vi "ShowMSStatus.vi"() -> ()   [LabVIEW 2015]
doc: "Use this template to create an application that executes until you click the Stop button. Unlike the Single Loop Application VI that uses polling, this VI uses the Event structure."
uses:
  _Server Global.vi
  Configuration/_Global Configuration.vi
panel:
  in  "Calibration":bool
  in  "ContactClosures":bool
  out "HideBox":bool
  in  "User Command":u16(ring)=7 items=["Start Run"=3, "Start Actual Run"=4, "Stop Run"=5, "Runtime Update"=6, "Get Data"=7, "Get Status"=8, "Get Table"=9, "Adv. Set Table"=10, "Get Configuration"=11, "Get Memory Map"=13, "Read ADC"=14, "Adv. Set Oscillator"=15, "Adv. Reboot Firmware"=16, "Adv. Backup Firmware"=17, "Adv. Update Firmware"=18, "Auxiliary Update"=19, "System Status"=20, "Start System"=21, "Shutdown System"=22, "Start LC Equilibration"=23, "Get LC Status"=24, "Get LC Configuration"=25, "Get LC Method Contents"=26, "Rinse Autosampler"=27, "Pump OnOff"=28, "Oven OnOff"=29, "Get LC Error"=30, "Clear LC Error"=31, "Set LC Input Logic"=32, "Set LC Hold Logic"=33, "Connect LC"=35, "Disconnect LC"=36]
  out "Corona Discharge:":sgl format="%.1f"
  out "ElectroSpray V2:":sgl
  out "ElectroSpray V1:":sgl
  in  "UpdateDisplay":bool
  out "Heating Gas 2:":sgl
  out "Heating Gas 1:":sgl
  out "Nebulizer Gas 1:":sgl
  out "Nebulizer Gas 2:":sgl
  out "Collision Pressure:":sgl format="%.1f"
  out "Dry Gas:":sgl
  out "Exhaust:":sgl
  out "Pump Speed:":sgl
  out "Exhaust OK":bool
  out "CurGas OK":bool
  out "Pump OK":bool
  out "Interlock OK":bool
  out "Vac. Pressure:":sgl format="%.2e"
  out "HSID Temp:":sgl
  out "Source 2 Temp:":sgl
  out "Source 2 Type:":i8(ring) items=["None", "ESI", "APCI", "APPI", "MicroSpray"]
  out "Source 1 Temp:":sgl
  out "Source 1 Type:":i8(ring) items=["None", "ESI", "APCI", "APPI", "MicroSpray"]
  out "Scans":i32 caption="Data Queue"
  out "Connected":bool=TRUE
  out "Error":string
  out "Data":string
  out "Ready":bool=TRUE
  in  "Message":string="<Method>\n  1\t0\t0\n  <Experiment>\n    1\t0\t0\t200\t0\t100\t1\t0\n    <MassRange>\n      200.000000\t400\t0.100000\t2000\t0.1\t0\n      <ParamTable/>\n    </MassRange>\n  </Experiment>\n</Method>"
  out "Data Queue":i32
  out "Busy":bool
  out "Locked":bool
  # "Source 1"
  # "Common Interface"
  # "Source 2"
  # "Other Status"
  # "Torr"
  # "Interlocks:"
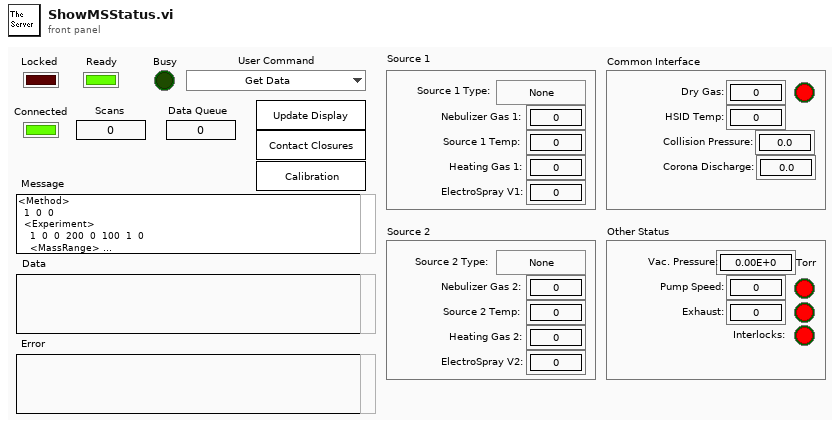
[diagram p1: front panel]
types:
  T1 = typedef "_Brief Status.ctl" = cluster{"Source 1 Type: ":T2, "Nebulizer Gas 1:":sgl, "Probe Temp 1: ":sgl, "Heating Gas 1:":sgl, "Source 2 Type:  ":T2, "Nebulizer Gas 2:":sgl, "Probe Temp 2: ":sgl, "Heating Gas 2:":sgl, "Dry Gas:":sgl, "HSID Temp:  ":sgl, "Collision Gas:":sgl, "Vac. Pressure: ":sgl, "Pump Speed:":sgl, "Exhaust:":sgl, "Interlock OK":bool, "CurGas OK":bool, "Pump OK":bool, "Exhaust OK":bool, "Event":string, "Corona Discharge:":sgl, "Source 1 Voltage:":sgl, "Source 2 Voltage:":sgl}
  T2 = typedef "_Source Type.ctl" = i8
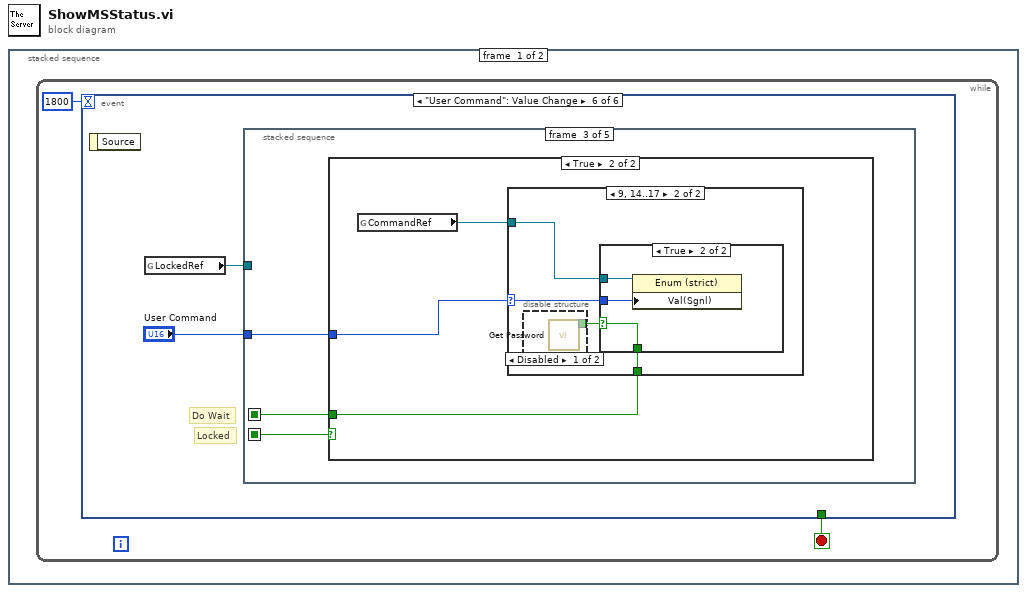
[diagram p0: block diagram]
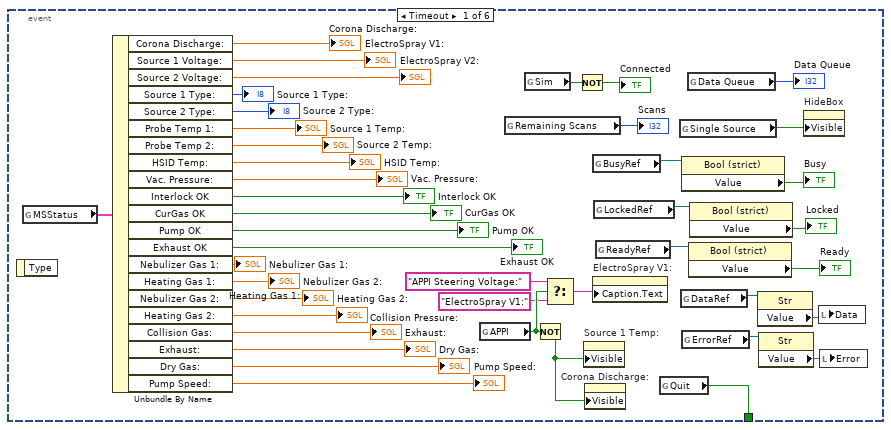
[diagram p2: hidden frame]
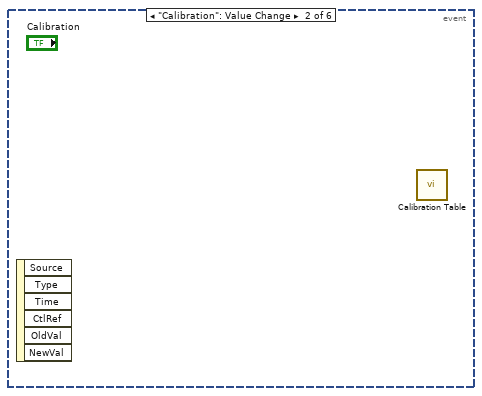
[diagram p3: hidden frame]
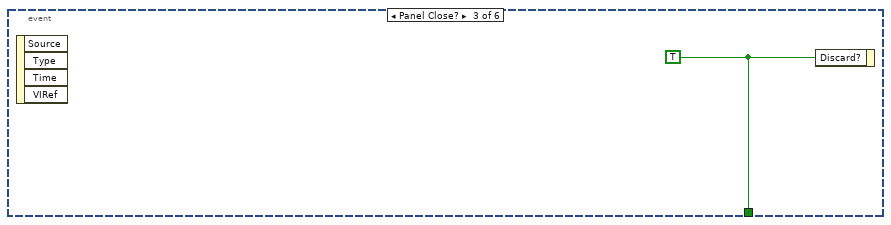
[diagram p4: hidden frame]
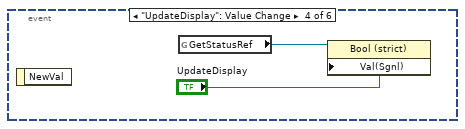
[diagram p5: hidden frame]
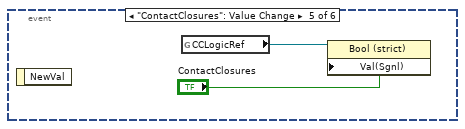
[diagram p6: hidden frame]
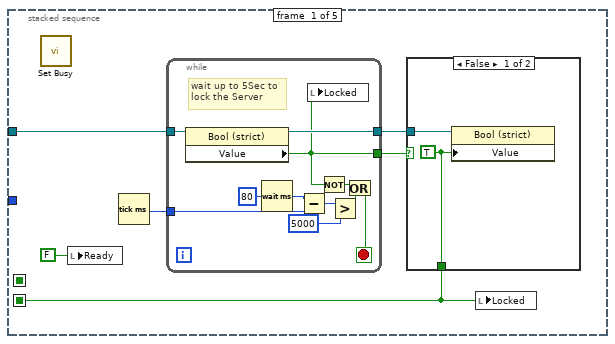
[diagram p7: hidden frame]
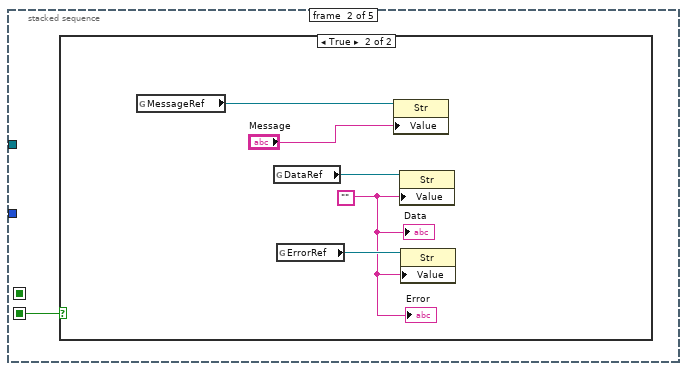
[diagram p9: hidden frame]
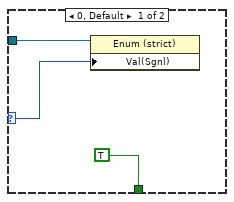
[diagram p12: hidden frame]
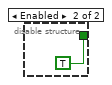
[diagram p13: hidden frame]
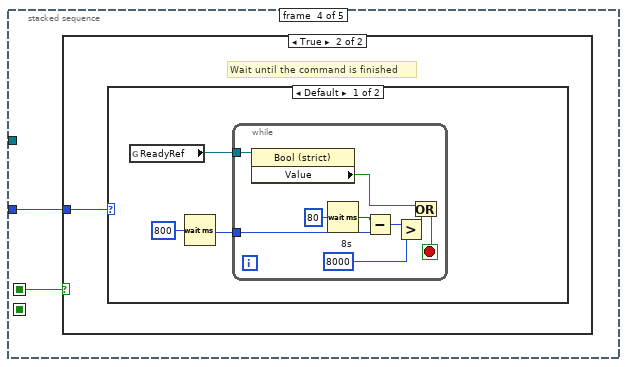
[diagram p15: hidden frame]
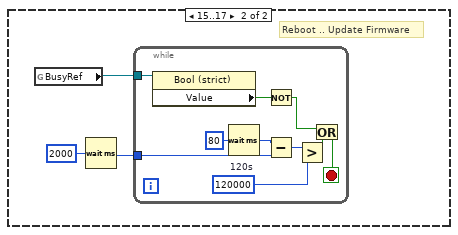
[diagram p17: hidden frame]
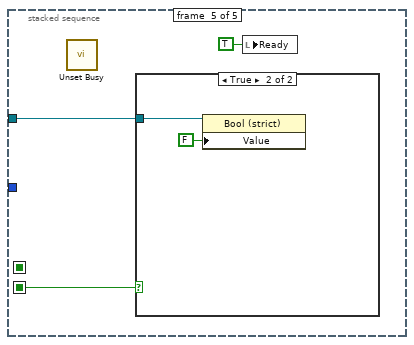
[diagram p18: hidden frame]
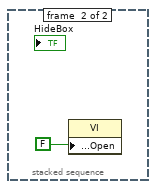
[diagram p20: hidden frame]
diagram:
  n1 = stacked-sequence {
    frame #0 {
      n2 = while {
        stop <- w1 stop-if-true
        n3 = event shown="[5] \"User Command\": Value Change" {
          selector: _ -> [_ _ _ _ _ _]
          dyn-events: _ -> [_ _ _ _ _ _]
          timeout: 1800 -> [_ _ _ _ _ _]
          tunnel: [w8 _ w46 _ _ _] -> w1
          event Timeout {
            n4 = event-data() -> ()  [unwired: 2 out]
            n5 = global read "_Server Global.vi" "MSStatus"() -> (w23:T1)
            n6 = Unbundle By Name(w23) -> ("Corona Discharge:"=→"Corona Discharge:":sgl, "Source 1 Voltage:"=→"ElectroSpray V1:":sgl, "Source 2 Voltage:"=→"ElectroSpray V2:":sgl, "Source 1 Type:"=→"Source 1 Type:":T2, "Source 2 Type:"=→"Source 2 Type:":T2, "Probe Temp 1:"=→"Source 1 Temp:":sgl, "Probe Temp 2:"=→"Source 2 Temp:":sgl, "HSID Temp:"=→"HSID Temp:":sgl, "Vac. Pressure:"=→"Vac. Pressure:":sgl, "Interlock OK"=→"Interlock OK":bool, "CurGas OK"=→"CurGas OK":bool, "Pump OK"=→"Pump OK":bool, "Exhaust OK"=→"Exhaust OK":bool, "Nebulizer Gas 1:"=→"Nebulizer Gas 1:":sgl, "Heating Gas 1:"=→"Heating Gas 1:":sgl, "Nebulizer Gas 2:"=→"Nebulizer Gas 2:":sgl, "Heating Gas 2:"=→"Heating Gas 2:":sgl, "Collision Gas:"=→"Collision Pressure:":sgl, "Exhaust:"=→"Exhaust:":sgl, "Dry Gas:"=→"Dry Gas:":sgl, "Pump Speed:"=→"Pump Speed:":sgl)
            n7 = global read "_Server Global.vi" "APPI"() -> (w6:bool)
            n8 = global read "_Server Global.vi" "Remaining Scans"() -> (→"Scans":i32)
            n9 = global read "_Global Configuration.vi" "Sim"() -> (w21:bool)
            n10 = Not(x=w6) -> (.not. x?=w7:bool)
            n11 = Select(t="APPI Steering Voltage:", s=w6, f="ElectroSpray V1:") -> (s? t:f=w3:string)
            n12 = Not(x=w21) -> (.not. x?=→"Connected":bool)
            n13 = property on="Source 1 Temp:" class="DigNum (strict)"("Visible"=w7) -> ()  [unwired: 2 in, 2 out]
            n14 = property on="Corona Discharge:" class="DigNum (strict)"("Visible"=w7) -> ()  [unwired: 2 in, 2 out]
            n15 = global read "_Server Global.vi" "BusyRef"() -> (w18:refnum<vi>)
            n16 = property on="ElectroSpray V1:" class="DigNum (strict)"("Caption.Text"=w3) -> ()  [unwired: 2 in, 2 out]
            n17 = global read "_Server Global.vi" "LockedRef"() -> (w16:refnum<vi>)
            n18 = global read "_Server Global.vi" "ReadyRef"() -> (w15:refnum<vi>)
            n19 = global read "_Global Configuration.vi" "Quit"() -> (w8:bool)
            n20 = global read "_Global Configuration.vi" "Single Source"() -> (w22:bool)
            n21 = global read "_Server Global.vi" "DataRef"() -> (w12:refnum<vi>)
            n22 = property class="Bool (strict)"(reference=w18) -> ("Value"=→"Busy":bool)  [unwired: 1 in, 2 out]
            n23 = global read "_Server Global.vi" "ErrorRef"() -> (w11:refnum<vi>)
            n24 = global read "_Server Global.vi" "Data Queue"() -> (→"Data Queue":i32)
            n25 = property class="Bool (strict)"(reference=w15) -> ("Value"=→"Ready":bool)  [unwired: 1 in, 2 out]
            n26 = property class="Bool (strict)"(reference=w16) -> ("Value"=→"Locked":bool)  [unwired: 1 in, 2 out]
            n27 = property class="Str"(reference=w12) -> ("Value"=w10:string)  [unwired: 1 in, 2 out]
            n28 = property class="Str"(reference=w11) -> ("Value"=w9:string)  [unwired: 1 in, 2 out]
            n29 = property on="HideBox" class="Bool (strict)"("Visible"=w22) -> ()  [unwired: 2 in, 2 out]
            n30 = local write "Data"(w10) -> ()
            n31 = local write "Error"(w9) -> ()
          }
          event "Calibration": Value Change {
            n32 = event-data() -> ()  [unwired: 7 out]
            n33 = call "Calibration Table.vi"() -> ()  [unwired: 4 in]
          }
          event Panel Close? {
            w46 = TRUE
            n34 = event-data() -> ()  [unwired: 5 out]
            n35 = event-data("Discard?"=w46) -> ()  [unwired: 1 in, 1 out]
          }
          event "UpdateDisplay": Value Change {
            n36 = event-data() -> ()  [unwired: 2 out]
            n37 = global read "_Server Global.vi" "GetStatusRef"() -> (w48:refnum<vi>)
            n38 = property class="Bool (strict)"(reference=w48, "Val(Sgnl)"="UpdateDisplay") -> ()  [unwired: 1 in, 2 out]
          }
          event "ContactClosures": Value Change {
            n39 = event-data() -> ()  [unwired: 2 out]
            n40 = global read "_Server Global.vi" "CCLogicRef"() -> (w50:refnum<vi>)
            n41 = property class="Bool (strict)"(reference=w50, "Val(Sgnl)"="ContactClosures") -> ()  [unwired: 1 in, 2 out]
          }
          event "User Command": Value Change {
            # "Do Wait"
            # "Locked"
            n42 = event-data() -> ()  [unwired: 2 out]
            n43 = global read "_Server Global.vi" "LockedRef"() -> (w52:refnum<vi>)
            n44 = stacked-sequence {
              seq-local: [w54 _ _ _ _] -> [_ w72 w80 _ w125]
              seq-local: [_ _ w78 _ _] -> [_ _ _ w97 _]
              tunnel: w52 -> [w55 _ _ _ w124]
              tunnel: "User Command" -> [_ _ w79 w96 _]
              frame #0 {
                n45 = call <vilib>:"Set Busy.vi"() -> ()  [unwired: 10 in, 2 out]
                n46 = local write "Ready"(FALSE ("Locked")) -> ()
                n47 = Tick Count (ms)() -> (millisecond timer value=w58:u32)
                n48 = while {
                  tunnel: [w61] -> w57
                  tunnel: w58 -> [w69]
                  tunnel: w55 -> [w63]
                  tunnel: [w62] -> w56
                  stop <- w64 stop-if-true
                  # "wait up to 5Sec to\nlock the Server"
                  n49 = property class="Bool (strict)"(reference=w63) -> (reference out=w62:refnum<vi>, "Value"=w61:bool)  [unwired: 1 in, 1 out]
                  n50 = Wait (ms)(milliseconds to wait=u32 80) -> (millisecond timer value=w70:u32)
                  n51 = Subtract(x=w70, y=w69) -> (x-y=w68:u32)
                  n52 = local write "Locked"(w61) -> ()
                  n53 = Not(x=w61) -> (.not. x?=w66:bool)
                  n54 = Greater?(x=w68, y=u32 5000) -> (0:w65:bool)
                  n55 = Or(x=w66, y=w65) -> (x .or. y?=w64:bool)
                }
                n56 = case shown="False" w57 {
                  tunnel: w56 -> [w60 _]
                  tunnel: [w59 _] -> w54
                  frame False {
                    w59 = TRUE ("Value")
                    n57 = property class="Bool (strict)"(reference=w60, "Value"=w59) -> ()  [unwired: 1 in, 2 out]
                  }
                  frame True {
                  }
                }
                n58 = local write "Locked"(w54) -> ()
              }
              frame #1 {
                n59 = case shown="True" w72 {
                  frame False {
                  }
                  frame True {
                    w73 = ""
                    n60 = global read "_Server Global.vi" "MessageRef"() -> (w77:refnum<vi>)
                    n61 = global read "_Server Global.vi" "DataRef"() -> (w75:refnum<vi>)
                    n62 = global read "_Server Global.vi" "ErrorRef"() -> (w74:refnum<vi>)
                    n63 = property class="Str"(reference=w77, "Value"="Message") -> ()  [unwired: 1 in, 2 out]
                    n64 = property class="Str"(reference=w75, "Value"=w73) -> ()  [unwired: 1 in, 2 out]
                    n65 = property class="Str"(reference=w74, "Value"=w73) -> ()  [unwired: 1 in, 2 out]
                    "Error" <- w73
                    "Data" <- w73
                  }
                }
              }
              frame #2 {
                n66 = case shown="True" w80 {
                  tunnel: w79 -> [_ w82]
                  tunnel: [_ w81] -> w78
                  frame False {
                  }
                  frame True {
                    n67 = global read "_Server Global.vi" "CommandRef"() -> (w83:refnum<vi>)
                    n68 = case shown="9, 14..17" w82 {
                      selector: w82 -> [w85 w89]
                      tunnel: w83 -> [w86 w88]
                      tunnel: [TRUE w87] -> w81
                      frame 0, Default {
                        n69 = property class="Enum (strict)"(reference=w86, "Val(Sgnl)"=w85) -> ()  [unwired: 1 in, 2 out]
                      }
                      frame 9, 14..17 {
                        n70 = disable-structure shown="Disabled" {
                          disable-tunnel: [w91 TRUE ("Valid")] -> w90
                          frame Disabled {
                            n71 = call "Get Password.vi"() -> ("Valid"=w91:bool)  [unwired: 1 in, 6 out]
                          }
                          frame Enabled {
                          }
                        }
                        n72 = case shown="True" w90 {
                          selector: w90 -> [_ w94]
                          tunnel: w89 -> [_ w93]
                          tunnel: w88 -> [_ w95]
                          tunnel: [_ w94] -> w87
                          frame False {
                          }
                          frame True {
                            n73 = property class="Enum (strict)"(reference=w95, "Val(Sgnl)"=w93) -> ()  [unwired: 1 in, 2 out]
                          }
                        }
                      }
                    }
                  }
                }
              }
              frame #3 {
                n74 = case shown="True" w97 {
                  tunnel: w96 -> [_ w98]
                  frame False {
                  }
                  frame True {
                    # "Wait until the command is finished"
                    n75 = case shown="Default" w98 {
                      frame Default {
                        n76 = global read "_Server Global.vi" "ReadyRef"() -> (w100:refnum<vi>)
                        n77 = Wait (ms)(milliseconds to wait=u32 800) -> (millisecond timer value=w101:u32)
                        n78 = while {
                          tunnel: w101 -> [w108]
                          tunnel: w100 -> [w103]
                          stop <- w104 stop-if-true
                          w106 = u32 8000  # 8s
                          n79 = property class="Bool (strict)"(reference=w103) -> ("Value"=w102:bool)  [unwired: 1 in, 2 out]
                          n80 = Wait (ms)(milliseconds to wait=u32 80) -> (millisecond timer value=w109:u32)
                          n81 = Subtract(x=w109, y=w108) -> (x-y=w107:u32)
                          n82 = Greater?(x=w107, y=w106) -> (0:w105:bool)
                          n83 = Or(x=w102, y=w105) -> (x .or. y?=w104:bool)
                        }
                      }
                      frame 15..17 {
                        # "Reboot .. Update Firmware"
                        n84 = global read "_Server Global.vi" "BusyRef"() -> (w112:refnum<vi>)
                        n85 = Wait (ms)(milliseconds to wait=u32 2000) -> (millisecond timer value=w113:u32)
                        n86 = while {
                          tunnel: w113 -> [w121]
                          tunnel: w112 -> [w116]
                          stop <- w117 stop-if-true
                          w119 = u32 120000  # 120s
                          n87 = property class="Bool (strict)"(reference=w116) -> ("Value"=w115:bool)  [unwired: 1 in, 2 out]
                          n88 = Wait (ms)(milliseconds to wait=u32 80) -> (millisecond timer value=w122:u32)
                          n89 = Not(x=w115) -> (.not. x?=w114:bool)
                          n90 = Subtract(x=w122, y=w121) -> (x-y=w120:u32)
                          n91 = Greater?(x=w120, y=w119) -> (0:w118:bool)
                          n92 = Or(x=w114, y=w118) -> (x .or. y?=w117:bool)
                        }
                      }
                    }
                  }
                }
              }
              frame #4 {
                n93 = call <vilib>:"Unset Busy.vi"() -> ()  [unwired: 11 in, 1 out]
                n94 = case shown="True" w125 {
                  tunnel: w124 -> [_ w128]
                  frame False {
                  }
                  frame True {
                    n95 = property class="Bool (strict)"(reference=w128, "Value"=FALSE) -> ()  [unwired: 1 in, 2 out]
                  }
                }
                n96 = local write "Ready"(TRUE ("Ready")) -> ()
              }
            }
          }
        }
      }
    }
    frame #1 {
      n97 = property class="VI"("Front Panel.Open"=FALSE ("Front Panel Window:Open")) -> ()  [unwired: 2 in, 2 out]
    }
  }
